vi "ADSR.vi"(6 "Sampling info":cluster{"Fs":dbl, "#s":dbl}={"Fs"=1000.0, "#s"=1000.0} {"Fs" format="%.2p"}, 7 "Boolean":bool, 8 "R":i32(slide) scale=0.0..100.0, 9 "S":i32(slide) scale=0.0..100.0, 10 "D":i32(slide) scale=0.0..100.0, 11 "A":i32(slide) scale=0.0..100.0) -> (0 "R":dbl[](graph), 1 "S":dbl[](graph), 2 "D":dbl[](graph), 3 "A":dbl[](graph))   [LabVIEW 2019]
uses:
  <vilib>/Analysis/1siggen.llb/Ramp Pattern by Samples.vi
  <vilib>/Analysis/NI_AALBase.lvlib
panel:
  out "ADSR":dbl[](graph)
  in  "Time constant (ms)":dbl=10000.0 format="%#_13g"
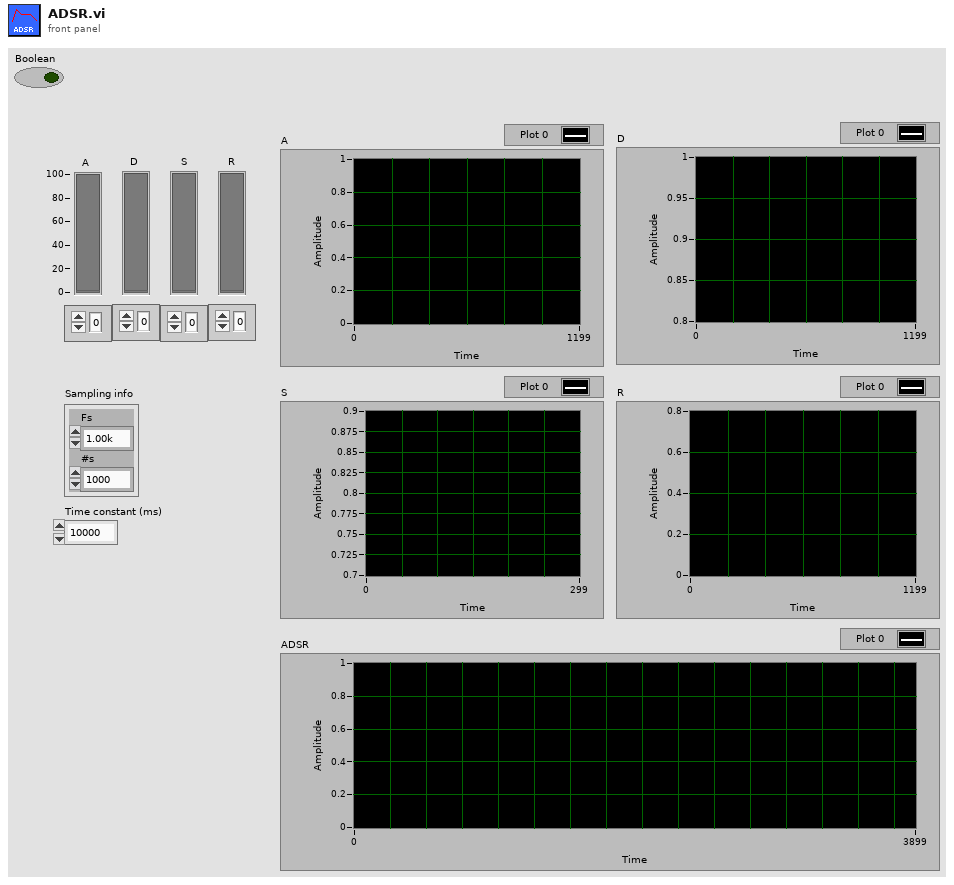
[diagram p1: front panel]
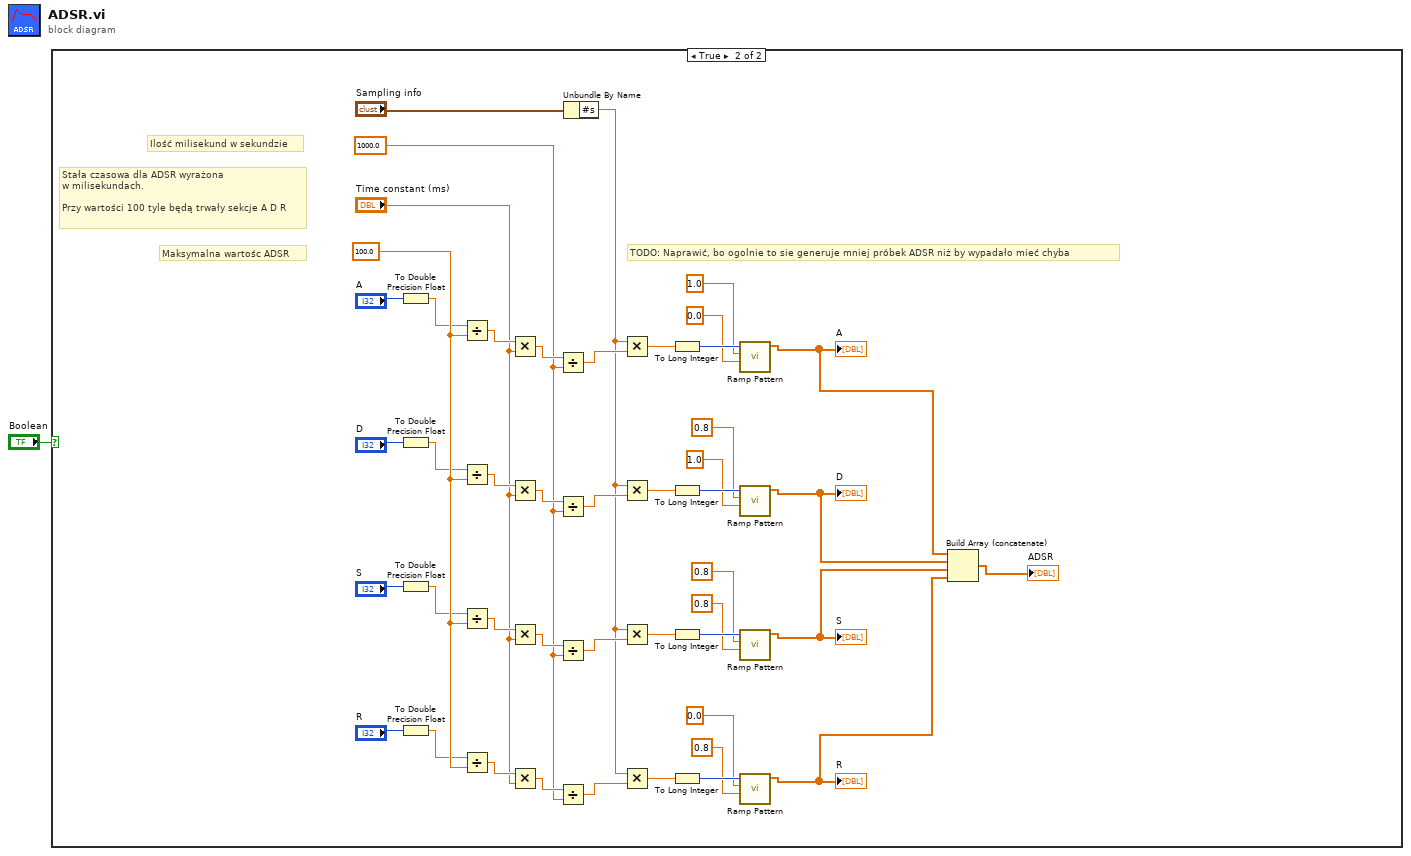
[diagram p0: block diagram]
diagram:
  n1 = case shown="True" "Boolean" {
    frame False {
    }
    frame True {
      w24 = 1000.0
      w47 = 100.0
      # "TODO: Naprawić, bo ogolnie to sie generuje mniej próbek ADSR niż by wypadało mieć chyba"
      # "Ilość milisekund w sekundzie"
      # "Maksymalna wartośc ADSR"
      # "Stała czasowa dla ADSR wyrażona\nw milisekundach.\n\nPrzy wartości 100 tyle będą trwały sekcje A D R"
      n2 = To Double Precision Float(number="A") -> (double precision float=w38:dbl)
      n3 = To Double Precision Float(number="D") -> (double precision float=w37:dbl)
      n4 = To Double Precision Float(number="S") -> (double precision float=w36:dbl)
      n5 = To Double Precision Float(number="R") -> (double precision float=w35:dbl)
      n6 = Divide(x=w38, y=w47) -> (x/y=w46:dbl)
      n7 = Divide(x=w37, y=w47) -> (x/y=w45:dbl)
      n8 = Divide(x=w36, y=w47) -> (x/y=w44:dbl)
      n9 = Divide(x=w35, y=w47) -> (x/y=w43:dbl)
      n10 = Multiply(x=w46, y="Time constant (ms)") -> (x*y=w33:dbl)
      n11 = Multiply(x=w45, y="Time constant (ms)") -> (x*y=w27:dbl)
      n12 = Multiply(x=w44, y="Time constant (ms)") -> (x*y=w26:dbl)
      n13 = Multiply(x=w43, y="Time constant (ms)") -> (x*y=w25:dbl)
      n14 = Divide(x=w33, y=w24) -> (x/y=w32:dbl)
      n15 = Divide(x=w27, y=w24) -> (x/y=w30:dbl)
      n16 = Divide(x=w26, y=w24) -> (x/y=w29:dbl)
      n17 = Divide(x=w25, y=w24) -> (x/y=w28:dbl)
      n18 = Unbundle By Name("Sampling info") -> ("#s"=w23:dbl)
      n19 = Multiply(x=w23, y=w32) -> (x*y=w22:dbl)
      n20 = Multiply(x=w23, y=w30) -> (x*y=w15:dbl)
      n21 = Multiply(x=w23, y=w29) -> (x*y=w7:dbl)
      n22 = Multiply(x=w23, y=w28) -> (x*y=w8:dbl)
      n23 = To Long Integer(number=w22) -> (32bit integer=w21:i32)
      n24 = To Long Integer(number=w15) -> (32bit integer=w18:i32)
      n25 = To Long Integer(number=w7) -> (32bit integer=w14:i32)
      n26 = To Long Integer(number=w8) -> (32bit integer=w11:i32)
      n27 = call-poly <vilib>:"Ramp Pattern.vi"("start"=0.0, "end"=1.0, "samples"=w21) -> ("Ramp Pattern"=w6:dbl[])  [unwired: 7 in, 1 out]
      "A" <- w6
      n28 = call-poly <vilib>:"Ramp Pattern.vi"("start"=1.0, "end"=0.8, "samples"=w18) -> ("Ramp Pattern"=w5:dbl[])  [unwired: 7 in, 1 out]
      "D" <- w5
      n29 = call-poly <vilib>:"Ramp Pattern.vi"("start"=0.8, "end"=0.8, "samples"=w14) -> ("Ramp Pattern"=w4:dbl[])  [unwired: 7 in, 1 out]
      "S" <- w4
      n30 = call-poly <vilib>:"Ramp Pattern.vi"("start"=0.8, "end"=0.0, "samples"=w11) -> ("Ramp Pattern"=w3:dbl[])  [unwired: 7 in, 1 out]
      "R" <- w3
      n31 = Build Array (concatenate)(w6, w5, w4, w3) -> (→"ADSR":dbl[])
    }
  }
